vi "basic-dependency-test.vi"(8 "error in (no error)":errorcluster) -> (0 "error out":errorcluster)   [LabVIEW 2021]
uses:
  <vilib>/addons/_JKI Toolkits/Caraya/classes/Test/Test.lvclass
  src/SMO/SMO.lvclass
  <vilib>/addons/_JKI Toolkits/Caraya/classes/Assert/Assert.lvclass
  src/SMO/Typedefs/SMOState --Enum.ctl
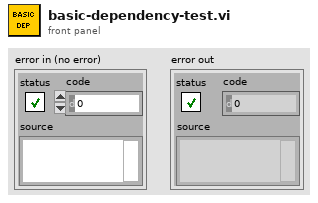
[diagram p1: front panel]
types:
  T1 = typedef "smo.lvlib/SMO.lvclass/SMOState --Enum.ctl" = enum16{"unknown", "Created", "Started", "Stopped"}
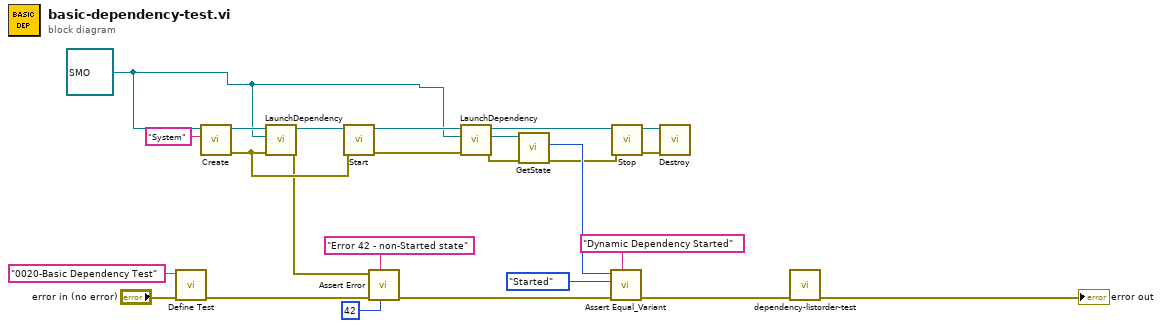
[diagram p0: block diagram]
diagram:
  w1 = refnum<class "SMO.lvclass"> refnum ("Dependency Type")
  n1 = call <vilib>:"Define Test.vi"("error in (no error)"="error in (no error)", "Label (VI Title)"="0020-Basic Dependency Test") -> ("error out"=w18:errorcluster)  [unwired: 9 in]
  n2 = call "Create.vi"("Subsystem Name (optional)"="System", "SMO"=w1) -> ("error out"=w15:errorcluster, "SMO out"=w22:refnum<class "SMO.lvclass">)  [unwired: 7 in, 1 out]
  n3 = call "LaunchDependency.vi"("error in (no error)"=w15, "Dependency Type"=w1, "SMO in"=w22) -> ("error out"=w14:errorcluster, "SMO out"=w21:refnum<class "SMO.lvclass">)  [unwired: 5 in, 2 out]
  n4 = call "Start.vi"("error in (no error)"=w15, "SMO"=w21) -> ("error out"=w12:errorcluster, "SMO out"=w13:refnum<class "SMO.lvclass">)  [unwired: 8 in]
  n5 = call <vilib>:"Assert Error.vi"("error code (1)"=42, "Label"="Error 42 - non-Started state", "error in (no error)"=w18, "Error?"=w14) -> ("error out"=w8:errorcluster)  [unwired: 7 in]
  n6 = call "LaunchDependency.vi"("error in (no error)"=w12, "Dependency Type"=w1, "SMO in"=w13) -> ("error out"=w9:errorcluster, "Dependency Reference"=w10:refnum<class "SMO.lvclass">, "SMO out"=w11:refnum<class "SMO.lvclass">)  [unwired: 5 in, 1 out]
  n7 = call "GetState.vi"("error in (no error)"=w9, "SMO"=w10) -> ("error out"=w4:errorcluster, "SMO State"=w7:T1)  [unwired: 7 in, 1 out]
  n8 = call <vilib>:"Assert Equal_Variant.vi"("Label"="Dynamic Dependency Started", "error in (no error)"=w8, "Y"=SMOState_--Enum."Started" ("SMO State"), "X"=w7) -> ("error out"=w3:errorcluster)  [unwired: 7 in]
  n9 = call "Stop.vi"("error in (no error)"=w4, "SMO"=w11) -> ("error out"=w20:errorcluster, "SMO out"=w19:refnum<class "SMO.lvclass">)  [unwired: 8 in]
  n10 = call "Destroy.vi"("error in (no error)"=w20, "SMO"=w19) -> ()  [unwired: 9 in, 1 out]
  n11 = call "dependency-listorder-test.vi"("error in (no error)"=w3) -> ("error out"=→"error out":errorcluster)  [unwired: 10 in]
